vi "Read All.vi"(8 "error in (no error)":errorcluster, 11 "VISA resource name":refnum<visa-resource-name>) -> (0 "error out":errorcluster, 2 "Data String":string, 3 "VISA resource name out":refnum<visa-resource-name>)   [LabVIEW 2020, in "AWG.lvlib" / "Agilent 3352X Series.lvlib"]
doc: "Reads all data in the data buffer of the VISA resource."
uses:
  Agilent 3352X Series.lvlib
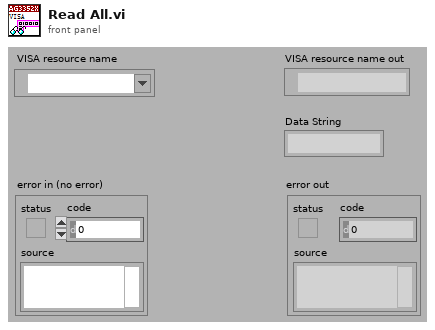
[diagram p1: front panel]
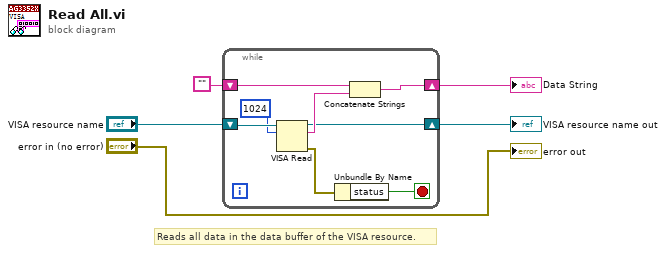
[diagram p0: block diagram]
diagram:
  # "Reads all data in the data buffer of the VISA resource."
  n1 = while {
    shift-right: [w7] -> w4
    shift-left: "" -> [w6]
    shift-right: [w9] -> w3
    shift-left: "VISA resource name" -> [w13]
    stop <- w12 stop-if-true
    n2 = VISA Read(VISA resource name=w13, byte count=u32 1024) -> (VISA resource name out=w9:refnum<visa-resource-name>, read buffer=w10:string, error out=w8:errorcluster)  [unwired: 1 in, 1 out]
    n3 = Unbundle By Name(w8) -> ("status"=w12:bool)
    n4 = Concatenate Strings(w6, w10) -> (w7:string)
  }
  "VISA resource name out" <- w3
  "Data String" <- w4
  "error out" <- "error in (no error)"
